vi "Area_Checkl_Main Function.vi"(0 "Image Src":T3, 5 "Rectangle":T2 {"Rotation" format="%.2f"; "Left" scale=0.0..1024.0; "Right" scale=0.0..1024.0}, 9 "Check Type":T1(ring), 11 "error in":errorcluster) -> (4 "Image Out":T3(plugin-control), 6 "%":dbl, 15 "error out":errorcluster)   [LabVIEW 2019]
uses:
  <vilib>/vision/Image Controls.llb/IMAQ Image.ctl
  <vilib>/vision/NI_Vision_Development_Module.lvlib
panel:
  out "Histogram":T4(graph)={"Starting Value"=2.5214942e-38, "Interval Width"=2.5214953e-38, "histogram"=[]}
  out "Gray Level Intensities":T5 {"Standard  Deviation" format="%.2f"; "Mean Intensity" format="%.2f"; "Maximum Intensity" format="%.2f"; "Minimum Intensity" format="%.2f"}
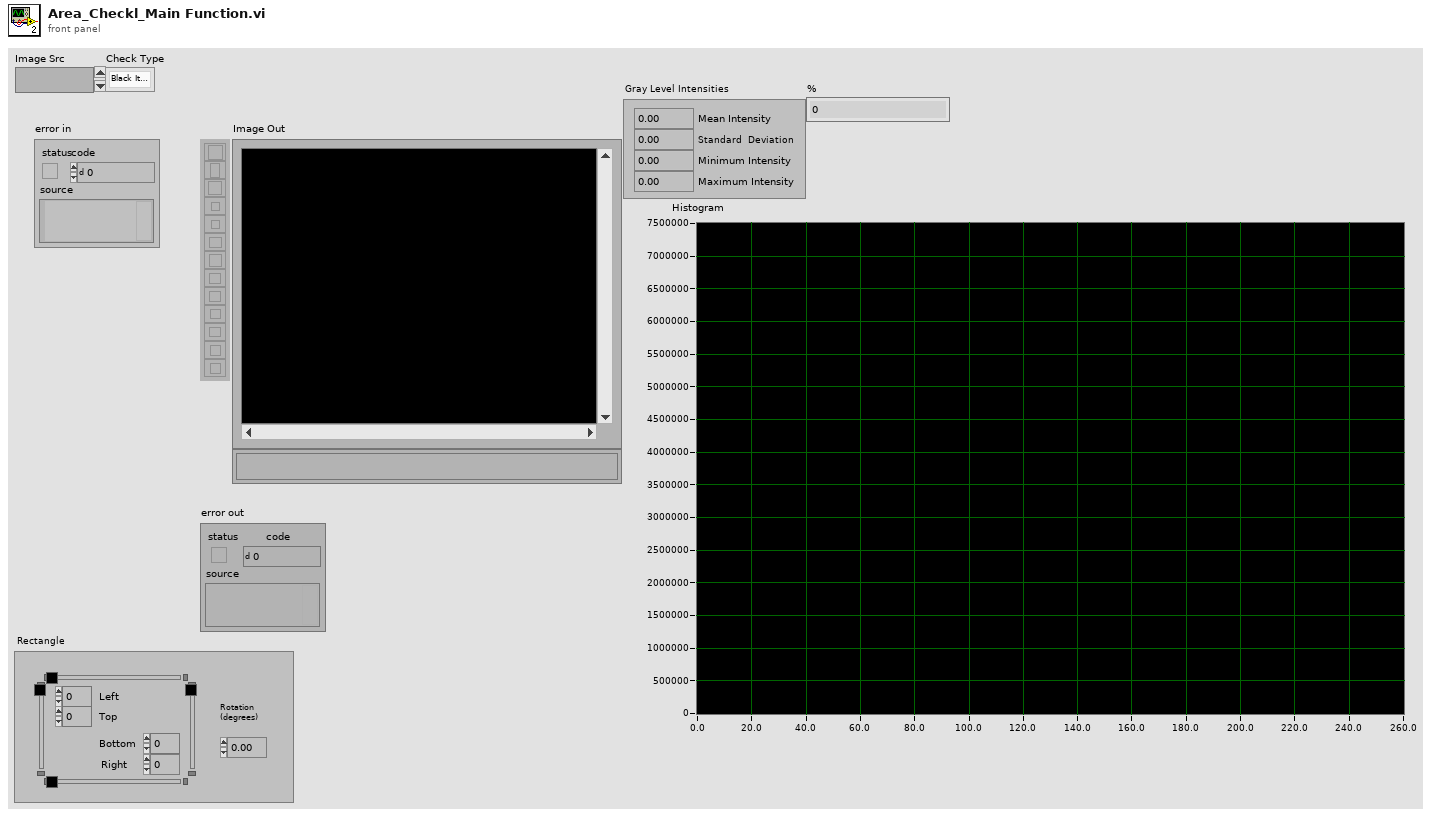
[diagram p1: front panel]
types:
  T1 = enum16{"Black Item White Ground", "White Item Black Ground"}
  T2 = typedef "IMAQ Rectangle" = cluster{"Left":i32, "Top":i32, "Right":i32, "Bottom":i32, "Rotation":dbl}
  T3 = typedef "IMAQ Image.ctl" = refnum<image>
  T4 = cluster{"Starting Value":sgl, "Interval Width":sgl, "histogram":u32[]}
  T5 = cluster{"Mean Intensity":sgl, "Standard  Deviation":sgl, "Minimum Intensity":sgl, "Maximum Intensity":sgl}
  T6 = typedef "Image Type" = u32
  T7 = cluster{"histogram":u32[], "Minimal Value":sgl, "Maximal Value":sgl, "Starting Value":sgl, "Interval Width":sgl, "Mean Value":sgl, "Standard  Variation":sgl, "Area (pixels)":i32}
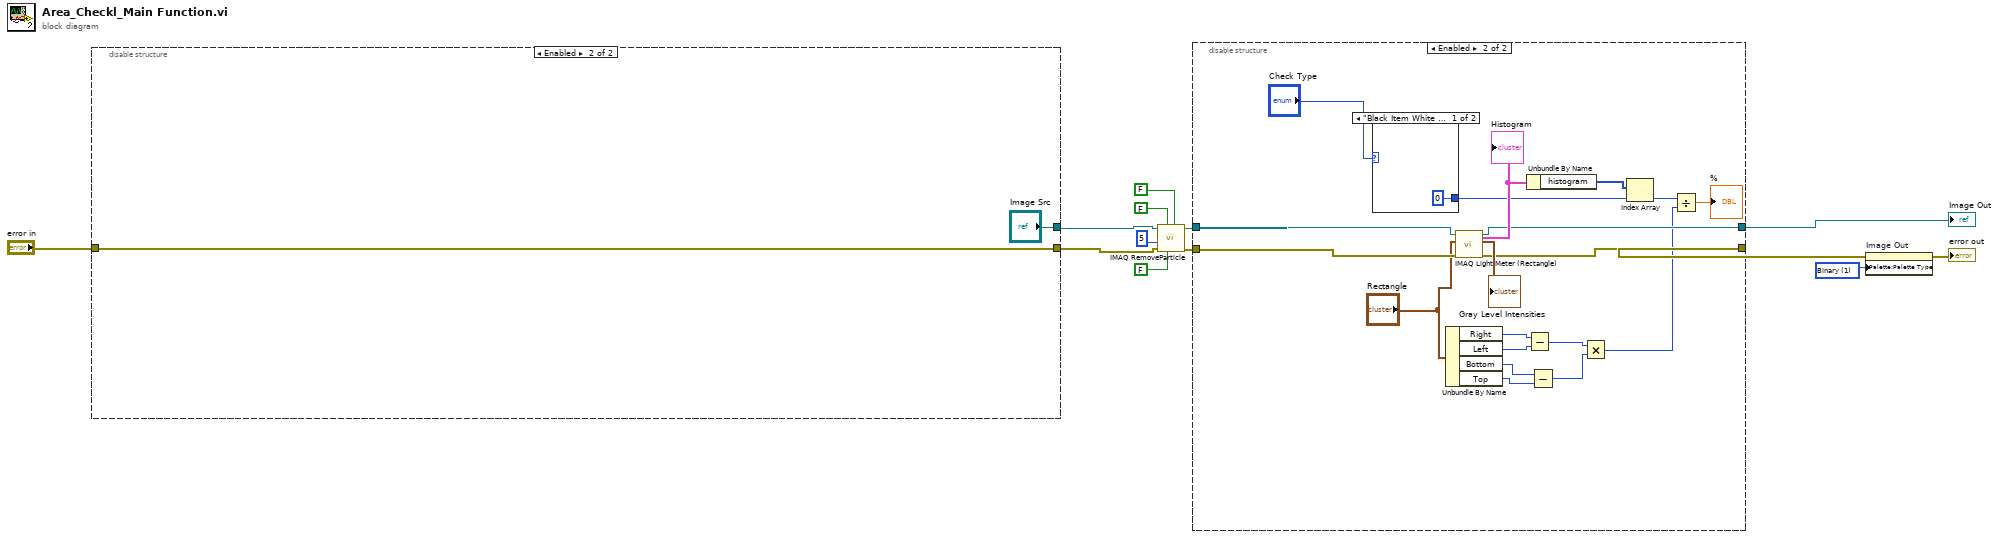
[diagram p0: block diagram]
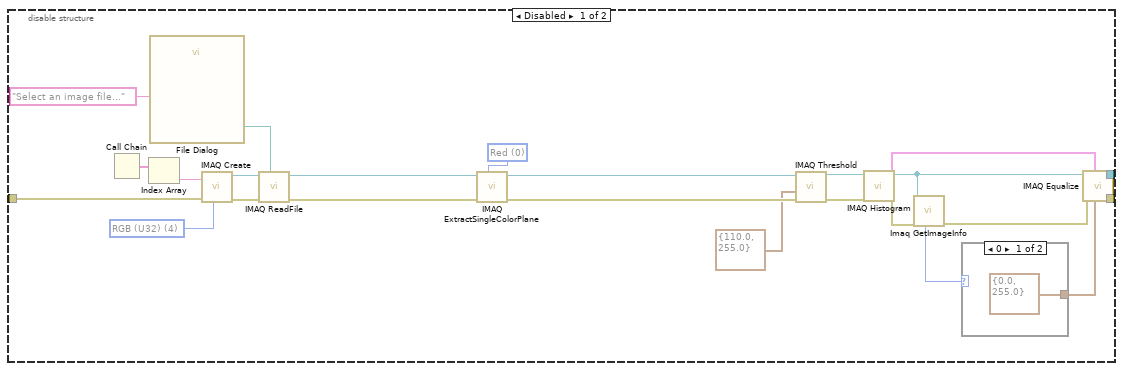
[diagram p2: hidden frame]
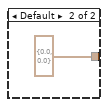
[diagram p3: hidden frame]
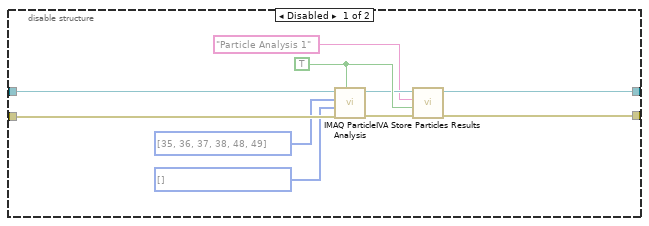
[diagram p4: hidden frame]
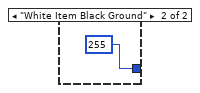
[diagram p5: hidden frame]
diagram:
  w3 = u32 1 items=["Grayscale", "Binary", "Gradient", "Rainbow", "Temperature", "User Defined", "Binary 16 Bit", "Gradient 16 Bit", "Rainbow 16 Bit", "Temperature 16 Bit", "User Defined 16 Bit"] ("Palette Type")
  n1 = disable-structure shown="Enabled" {
    disable-tunnel: "error in" -> [w33 w40]
    disable-tunnel: [w15 w40] -> w2
    disable-tunnel: [w14 "Image Src"] -> w1
    frame Disabled {
      w27 = 0 items=["Red", "Green", "Blue", "Hue", "Saturation", "Luminance", "Value", "Intensity"] ("Color Plane")
      w28 = T6 4 items=["Grayscale (U8)", "Grayscale (I16)", "Grayscale (SGL)", "Complex (CSG)", "RGB (U32)", "HSL (U32)", "RGB (U64)", "Grayscale (U16)"] ("Image Type")
      n2 = Call Chain() -> (call chain=w32:string[])
      n3 = Index Array(array=w32) -> (element=w31:string)  [unwired: 1 in]
      n4 = call "File Dialog"("prompt"="Select an image file...") -> ("selected path"=w29:path)  [unwired: 6 in, 8 out]
      n5 = call "IMAQ Create"("Image Name"=w31, "Image Type"=w28, "error in (no error)"=w33) -> ("New Image"=w35:T3, "error out"=w34:errorcluster)  [unwired: 1 in, 1 out]
      n6 = call "IMAQ ReadFile"("File Path"=w29, "error in (no error)"=w34, "Image"=w35) -> ("error out"=w36:errorcluster, "Image Out"=w26:T3)  [unwired: 2 in, 5 out]
      n7 = call "IMAQ ExtractSingleColorPlane"("Color Plane"=w27, "error in (no error)"=w36, "Image Src"=w26) -> ("error out"=w25:errorcluster, "Image Dst Out"=w23:T3)  [unwired: 1 in, 6 out]
      n8 = call "IMAQ Threshold"("error in (no error)"=w25, "Range"=cluster{"Lower value":sgl, "Upper value":sgl} {"Lower value"=110.0, "Upper value"=255.0}, "Image Src"=w23) -> ("error out"=w16:errorcluster, "Image Dst Out"=w17:T3)  [unwired: 3 in, 4 out]
      n9 = call "IMAQ Histogram"("error in (no error)"=w16, "Image"=w17) -> ("error out"=w20:errorcluster, "Histogram Report"=w22:T7)  [unwired: 3 in, 5 out]
      n10 = call "Imaq GetImageInfo"("error in (no error)"=w20, "Image"=w17) -> ("error out"=w19:errorcluster, "Image Type"=w21:T6)  [unwired: 8 out]
      n11 = case shown="0" w21 {
        tunnel: [cluster{"Minimum":sgl, "Maximum":sgl} {"Minimum"=0.0, "Maximum"=255.0} ("Range") cluster{"Minimum":sgl, "Maximum":sgl} {"Minimum"=0.0, "Maximum"=0.0} ("Range")] -> w18
        frame 0 {
        }
        frame Default {
        }
      }
      n12 = call "IMAQ Equalize"("Range"=w18, "Histogram Report"=w22, "error in (no error)"=w19, "Image Src"=w17) -> ("error out"=w15:errorcluster, "Image Dst Out"=w14:T3)  [unwired: 2 in, 4 out]
    }
    frame Enabled {
    }
  }
  n13 = call "IMAQ RemoveParticle"("Connectivity 4/8 (8)"=FALSE, "Low Pass/High Pass (Low)"=FALSE, "Square/Hexa (Square)"=FALSE, "error in (no error)"=w2, "Number of Erosion"=5, "Image Src"=w1) -> ("error out"=w8:errorcluster, "Image Dst Out"=w7:T3)  [unwired: 1 in, 3 out]
  n14 = disable-structure shown="Enabled" {
    disable-tunnel: w8 -> [w50 w66]
    disable-tunnel: w7 -> [w47 w69]
    disable-tunnel: [w42 w67] -> w6
    disable-tunnel: [w41 w61] -> w4
    frame Disabled {
      w48 = i32[] [] items=["Center of Mass X", "Center of Mass Y", "First Pixel X", "First Pixel Y", "Bounding Rect Left", "Bounding Rect Top", "Bounding Rect Right", "Bounding Rect Bottom", "Max Feret Diameter Start X", "Max Feret Diameter Start Y", "Max Feret Diameter End X", "Max Feret Diameter End Y", "Max Horiz. Segment Length Left", "Max Horiz. Segment Length Right", "Max Horiz. Segment Length Row", "-", "Bounding Rect Width", "Bounding Rect Height", "Bounding Rect Diagonal", "Perimeter", "Convex Hull Perimeter", "Holes' Perimeter", "Max Feret Diameter", "Equivalent Ellipse Major Axis", "Equivalent Ellipse Minor Axis", "Equivalent Ellipse Minor Axis (Feret)", "Equivalent Rect Long Side", "Equivalent Rect Short Side", "Equivalent Rect Diagonal", "Equivalent Rect Short Side (Feret)", "Average Horiz. Segment Length", "Average Vert. Segment Length", "Hydraulic Radius", "Waddel Disk Diameter", "-", "Area", "Holes' Area", "Particle & Holes' Area", "Convex Hull Area", "Image Area", "-", "Number of Holes", "Number of Horiz. Segments", "Number of Vert. Segments", "-", "Orientation", "Max Feret Diameter Orientation", "-", "% Area/Image Area", "% Area/(Particle & Holes' Area)", "Ratio of Equivalent Ellipse Axes", "Ratio of Equivalent Rect Sides", "-", "Elongation Factor", "Compactness Factor", "Heywood Circularity Factor", "Type Factor", "-", "Sum X", "Sum Y", "Sum XX", "Sum XY", "Sum YY", "Sum XXX", "Sum XXY", "Sum XYY", "Sum YYY", "-", "Moment of Inertia XX", "Moment of Inertia XY", "Moment of Inertia YY", "Moment of Inertia XXX", "Moment of Inertia XXY", "Moment of Inertia XYY", "Moment of Inertia YYY", "Norm. Moment of Inertia XX", "Norm. Moment of Inertia XY", "Norm. Moment of Inertia YY", "Norm. Moment of Inertia XXX", "Norm. Moment of Inertia XXY", "Norm. Moment of Inertia XYY", "Norm. Moment of Inertia YYY", "Hu Moment 1", "Hu Moment 2", "Hu Moment 3", "Hu Moment 4", "Hu Moment 5", "Hu Moment 6", "Hu Moment 7"] ("Real-World Measurements")
      w49 = i32[] [35, 36, 37, 38, 48, 49] items=["Center of Mass X", "Center of Mass Y", "First Pixel X", "First Pixel Y", "Bounding Rect Left", "Bounding Rect Top", "Bounding Rect Right", "Bounding Rect Bottom", "Max Feret Diameter Start X", "Max Feret Diameter Start Y", "Max Feret Diameter End X", "Max Feret Diameter End Y", "Max Horiz. Segment Length Left", "Max Horiz. Segment Length Right", "Max Horiz. Segment Length Row", "-", "Bounding Rect Width", "Bounding Rect Height", "Bounding Rect Diagonal", "Perimeter", "Convex Hull Perimeter", "Holes' Perimeter", "Max Feret Diameter", "Equivalent Ellipse Major Axis", "Equivalent Ellipse Minor Axis", "Equivalent Ellipse Minor Axis (Feret)", "Equivalent Rect Long Side", "Equivalent Rect Short Side", "Equivalent Rect Diagonal", "Equivalent Rect Short Side (Feret)", "Average Horiz. Segment Length", "Average Vert. Segment Length", "Hydraulic Radius", "Waddel Disk Diameter", "-", "Area", "Holes' Area", "Particle & Holes' Area", "Convex Hull Area", "Image Area", "-", "Number of Holes", "Number of Horiz. Segments", "Number of Vert. Segments", "-", "Orientation", "Max Feret Diameter Orientation", "-", "% Area/Image Area", "% Area/(Particle & Holes' Area)", "Ratio of Equivalent Ellipse Axes", "Ratio of Equivalent Rect Sides", "-", "Elongation Factor", "Compactness Factor", "Heywood Circularity Factor", "Type Factor", "-", "Sum X", "Sum Y", "Sum XX", "Sum XY", "Sum YY", "Sum XXX", "Sum XXY", "Sum XYY", "Sum YYY", "-", "Moment of Inertia XX", "Moment of Inertia XY", "Moment of Inertia YY", "Moment of Inertia XXX", "Moment of Inertia XXY", "Moment of Inertia XYY", "Moment of Inertia YYY", "Norm. Moment of Inertia XX", "Norm. Moment of Inertia XY", "Norm. Moment of Inertia YY", "Norm. Moment of Inertia XXX", "Norm. Moment of Inertia XXY", "Norm. Moment of Inertia XYY", "Norm. Moment of Inertia YYY", "Hu Moment 1", "Hu Moment 2", "Hu Moment 3", "Hu Moment 4", "Hu Moment 5", "Hu Moment 6", "Hu Moment 7"] ("Pixel Measurements")
      w46 = TRUE ("Connectivity 4/8 (8)")
      n15 = call "IMAQ Particle Analysis"("Connectivity 4/8 (8)"=w46, "error in (no error)"=w50, "Real-World Measurements"=w48, "Pixel Measurements"=w49, "Image"=w47) -> ("error out"=w43:errorcluster, "Image Out (duplicate)"=w45:T3)  [unwired: 5 out]
      n16 = call <vilib>:"IVA Store Particles Results.vi"("error in (no error)"=w43, "Connectivity 4/8 (8)"=w46, "Step Name"="Particle Analysis 1", "Image in"=w45) -> ("error out"=w42:errorcluster, "Image dup"=w41:T3)  [unwired: 6 out]
    }
    frame Enabled {
      n17 = case shown="\"Black Item White Ground\", Default" "Check Type" {
        tunnel: [0 ("index") 255 ("index")] -> w51
        frame "Black Item White Ground", Default {
        }
        frame "White Item Black Ground" {
        }
      }
      n18 = Unbundle By Name("Rectangle") -> ("Right"=w60:i32, "Left"=w59:i32, "Bottom"=w58:i32, "Top"=w57:i32)
      n19 = call "IMAQ Light Meter (Rectangle)"("error in (no error)"=w66, "Rectangle"="Rectangle", "Image"=w69) -> ("error out"=w67:errorcluster, "Gray Level Intensities"=→"Gray Level Intensities":T5, "Image Out"=w61:T3, "Histogram"=w65:T4)  [unwired: 4 in, 1 out]
      "Histogram" <- w65
      n20 = Unbundle By Name(w65) -> ("histogram"=w64:u32[])
      n21 = Subtract(x=w60, y=w59) -> (x-y=w56:i32)
      n22 = Subtract(x=w58, y=w57) -> (x-y=w55:i32)
      n23 = Multiply(x=w56, y=w55) -> (x*y=w54:i32)
      n24 = Index Array(array=w64, index=w51) -> (element=w63:u32)
      n25 = Divide(x=w63, y=w54) -> (x/y=→"%":dbl)
    }
  }
  "Image Out" <- w4
  n26 = property on="Image Out" class="ImageControl"(error in=w6, "Palette:Palette Type"=w3) -> (error out=→"error out":errorcluster)  [unwired: 1 in, 1 out]
